vi "Input.vi"() -> (3 "产品编号":string)   [LabVIEW 2017]
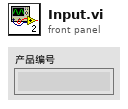
[diagram p1: front panel]
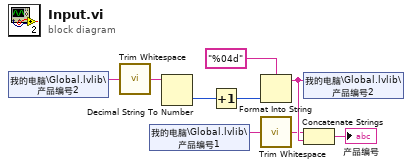
[diagram p0: block diagram]
diagram:
  n1 = shared-variable "我的电脑\\Global.lvlib\\产品编号2"() -> (w7:string)  [unwired: 1 in, 1 out]
  n2 = call <vilib>:"Trim Whitespace.vi"("string"=w7) -> ("trimmed string"=w6:string)  [unwired: 1 in]
  n3 = shared-variable "我的电脑\\Global.lvlib\\产品编号1"() -> (w2:string)  [unwired: 1 in, 1 out]
  n4 = Decimal String To Number(string=w6) -> (number=w9:i32)  [unwired: 2 in, 1 out]
  n5 = Increment(x=w9) -> (x+1=w4:i32)
  n6 = Format Into String(format string="%04d" ("格式字符串"), w4) -> (resulting string=w3:string)  [unwired: 2 in, 1 out]
  n7 = call <vilib>:"Trim Whitespace.vi"("string"=w2) -> ("trimmed string"=w1:string)  [unwired: 1 in]
  n8 = shared-variable "我的电脑\\Global.lvlib\\产品编号2"(w3) -> ()  [unwired: 1 in, 1 out]
  n9 = Concatenate Strings(w1, w3) -> (→"产品编号":string)
